vi "Edit Children Data.vi"(7 "Active Column Number":i32, 8 "Error In":errorcluster, 9 "String":string, 10 "Child Tag":string, 11 "Tree Reference In":refnum<vi>) -> (0 "Error out":errorcluster, 3 "Tree Reference Out":refnum<vi>)   [LabVIEW 2013, in "QuickVIew.lvlib"]
doc: "Collects and returns all tags of parents immediate children. If the parent tag is an empty string, the currently selected item is used."
uses:
  QuickVIew.lvlib
panel:
  # "VI INPUTS"
  # "VI OUTPUTS"
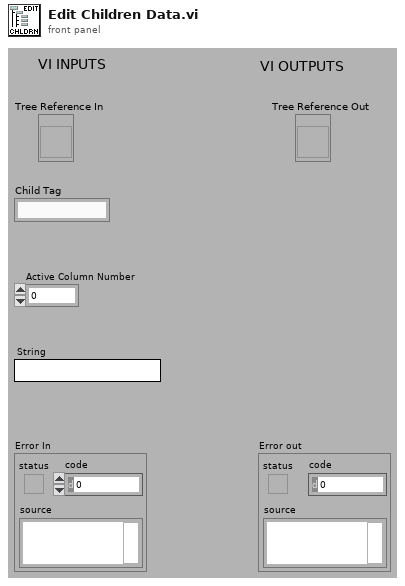
[diagram p1: front panel]
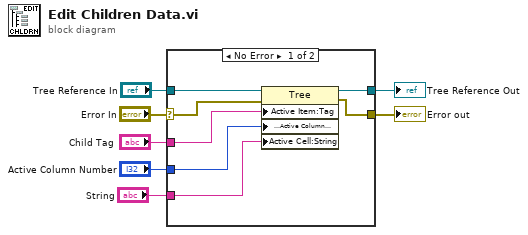
[diagram p0: block diagram]
diagram:
  n1 = case shown="No Error" "Error In" {
    selector: "Error In" -> [w13 w15]
    tunnel: "Tree Reference In" -> [w14 w16]
    tunnel: "Child Tag" -> [w12 _]
    tunnel: [w9 w16] -> w6
    tunnel: [w8 w15] -> w5
    tunnel: "Active Column Number" -> [w11 _]
    tunnel: "String" -> [w10 _]
    frame No Error {
      n2 = property class="Tree"(reference=w14, error in=w13, "Active Item:Tag"=w12, "Active Cell:Active Column Number"=w11, "Active Cell:String"=w10) -> (reference out=w9:refnum<vi>, error out=w8:errorcluster)
    }
    frame Error {
    }
  }
  "Tree Reference Out" <- w6
  "Error out" <- w5
